vi "Begin.vi"(8 "error in":errorcluster) -> (0 "error out":errorcluster)   [LabVIEW 2016]
doc: "Called before other user functions, this VI is expected to open initial I/O refnums, load in file data, and do all program initialization. Notice that the <B>error out</B> terminal is simply used for data flow. Wiring it to other structures or subVIs ensures that this VI runs first."
uses:
  <vilib>/Rock Robotics/WPI/SafetyOutput/WPI_SafetyOutputConfigMenu.ctl
  <vilib>/Rock Robotics/WPI/DriverStation/WPI_DriverStationRobotMode2.ctl
  <vilib>/Rock Robotics/WPI/Joystick/WPI_JoystickDeviceEnum.ctl
  <vilib>/Rock Robotics/SystemInterfaces/AI/FPGA_AIChannel.ctl
  <vilib>/Rock Robotics/SystemInterfaces/DIO/FPGA_DIOChannel.ctl
  <vilib>/Rock Robotics/SystemInterfaces/i2clib/i2c_bus.ctl
  <vilib>/Rock Robotics/SystemInterfaces/DIO/FPGA_DIOPWMChannel.ctl
  <vilib>/Rock Robotics/SystemInterfaces/DIO/FPGA_DIORelayChannel.ctl
  <vilib>/Rock Robotics/WPI/Relay/WPI_RelayDirection.ctl
  <vilib>/Rock Robotics/WPI/Solenoid/WPI_SolenoidChannel.ctl
  Libraries/TalonSRX/TalonSRX/WPI_CANTalonSRX_APIControlMode.ctl
  Libraries/TalonSRX/TalonSRX/WPI_CANTalonSRX_APIFeedbackSelect.ctl
  Robot Global Data.vi
  <vilib>/Rock Robotics/Network Tables/NT Write String Array.vi
  <vilib>/Rock Robotics/WPI/MotorControl/WPI_MotorControlOpen SPARK.vi
  <vilib>/Rock Robotics/WPI/Solenoid/WPI_SolenoidOpenDouble.vi
  <vilib>/Rock Robotics/WPI/RobotDrive/WPI_RobotDriveOpen2MotorWithExistingMotors.vi
  Libraries/navX Library v2/navX Library v2.lvlib
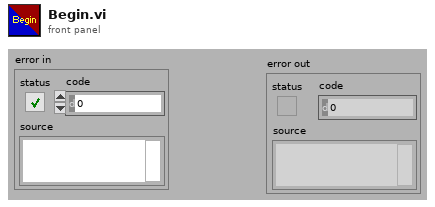
[diagram p1: front panel]
types:
  T1 = typedef "WPI_SolenoidChannel.ctl" = enum8{"Solenoid 0", "Solenoid 1", "Solenoid 2", "Solenoid 3", "Solenoid 4", "Solenoid 5", "Solenoid 6", "Solenoid 7", "Invalid"}
  T2 = typedef "WPI_CANTalonSRX_APIFeedbackSelect.ctl" = enum16{"Digital Quadrature Encoder", "Analog Potentiometer", "Analog Encoder", "Count on Quad-A (Rising-Edge)", "Count on Quad-A (Falling-Edge)", "CTR Magnetic Enc (Absolute)", "CTR Magnetic Enc (Relative)", "Pulse Width"}
  T3 = typedef "WPI_CANTalonSRX_APIControlMode.ctl" = enum8{"Percent VBus", "Speed", "Position", "Slave", "Unchanged / Invalid", "Voltage Compensation", "Current", "Motion Profile", "Motion Magic"}
  T4 = typedef "WPI_RelayDirection.ctl" = enum16{"Both directions", "Forward only", "Reverse only"}
  T5 = typedef "FPGA_DIORelayChannel.ctl" = enum8{"Relay 0", "Relay 1", "Relay 2", "Relay 3", "Invalid"}
  T6 = typedef "FPGA_DIOPWMChannel.ctl" = enum8{"PWM 0", "PWM 1", "PWM 2", "PWM 3", "PWM 4", "PWM 5", "PWM 6", "PWM 7", "PWM 8", "PWM 9", "PWM MXP 0", "PWM MXP 1", "PWM MXP 2", "PWM MXP 3", "PWM MXP 4", "PWM MXP 5", "PWM MXP 6", "PWM MXP 7", "PWM MXP 8", "PWM MXP 9", "Invalid"}
  T7 = typedef "FPGA_AIChannel.ctl" = enum8{"AI 0", "AI 1", "AI 2", "AI 3", "AI MXP 0", "AI MXP 1", "AI MXP 2", "AI MXP 3", "Invalid"}
  T8 = typedef "FPGA_DIOChannel.ctl" = enum8{"DIO 0", "DIO 1", "DIO 2", "DIO 3", "DIO 4", "DIO 5", "DIO 6", "DIO 7", "DIO 8", "DIO 9", "DIO MXP 0", "DIO MXP 1", "DIO MXP 2", "DIO MXP 3", "DIO MXP 4", "DIO MXP 5", "DIO MXP 6", "DIO MXP 7", "DIO MXP 8", "DIO MXP 9", "DIO MXP 10", "DIO MXP 11", "DIO MXP 12", "DIO MXP 13", "DIO MXP 14", "DIO MXP 15", "SPI Port CS1", "SPI Port CS2", "SPI Port CS3", "SPI Port MISO", "SPI Port MOSI", "Invalid"}
  T9 = typedef "WPI_JoystickDeviceEnum.ctl" = enum16{"USB 0", "USB 1", "USB 2", "USB 3", "USB 4", "USB 5"}
  T10 = typedef "i2c_bus.ctl" = enum16{"I2C On-Board", "I2C MXP", "Invalid"}
  T11 = typedef "WPI_DriverStationRobotMode2.ctl" = enum16{"Autonomous Disabled", "Autonomous Enabled", "Teleop Disabled", "Teleop Enabled", "Disconnected", "Finish", "Test Disabled", "Test Enabled", "Emergency Stopped"}
  T12 = typedef "WPI_SafetyOutputConfigMenu.ctl" = enum16{"Enable", "Disable"}
  T13 = typedef "WPI_MotorControlDeviceRef.ctl" = cluster{"DeviceStatus":errorcluster, "Type":T14, "PWM":cluster{"PWM Channel":T6, "DeadBand":T15}, "CAN":cluster{"Device Number":u8, "SetOutput VI Ref":variant, "GetOutput VI Ref":variant, "Enable VI Ref":variant, "Disable VI Ref":variant, "Data":variant}, "Invert":bool}
  T14 = typedef "WPI_MotorControlType.ctl" = enum16{"PWM", "CAN"}
  T15 = typedef "WPI_PWMDeadband.ctl" = cluster{"Name":string, "maxPositivePwm":i32, "minPositivePwm":i32, "centerPwm":i32, "maxNegativePwm":i32, "minNegativePwm":i32, "angularRange":u16}
  T16 = typedef "WPI_AnalogChannelDevRef.ctl" = cluster{"DevStatus":errorcluster, "Analog Channel":T7}
  T17 = typedef "WPI_DigitalInputDevRef.ctl" = cluster{"DevStatus":errorcluster, "DIO Channel":T8}
  T18 = typedef "WPI_JoystickDevRef.ctl" = cluster{"Device":T9}
  T19 = typedef "navX Library v2.lvlib/Z900_navX_DeviceTypeDef.ctl" = cluster{"Interface":cluster{"Protocol":T20, "Update Rate (4Hz-100Hz)":u8, "navX Open TypeDef":variant}, "Notify Packet":refnum<notifier>, "Loop VI Refnum":refnum<vi>, "Ready to Close Occurrence Refnum":refnum<k4>}
  T20 = typedef "navX Library v2.lvlib/Z900_navX_ProtocolTypeDef.ctl" = enum16{"SERIAL", "I2C", "SPI"}
  T21 = typedef "WPI_SolenoidDevRef.ctl" = cluster{"DevStatus":errorcluster, "Pneumatics Control Module":u8, "Forward Solenoid Channel":T1, "Reverse Solenoid Channel":T1}
  T22 = typedef "WPI_RelayDevRef.ctl" = cluster{"DevStatus":errorcluster, "Relay Channel":T5, "Relay Direction":T4}
  T23 = typedef "WPI_RobotDriveDevRef.ctl" = cluster{"DevStatus":errorcluster, "Motors[]":T13[], "Square Inputs":bool, "Max Output":dbl}
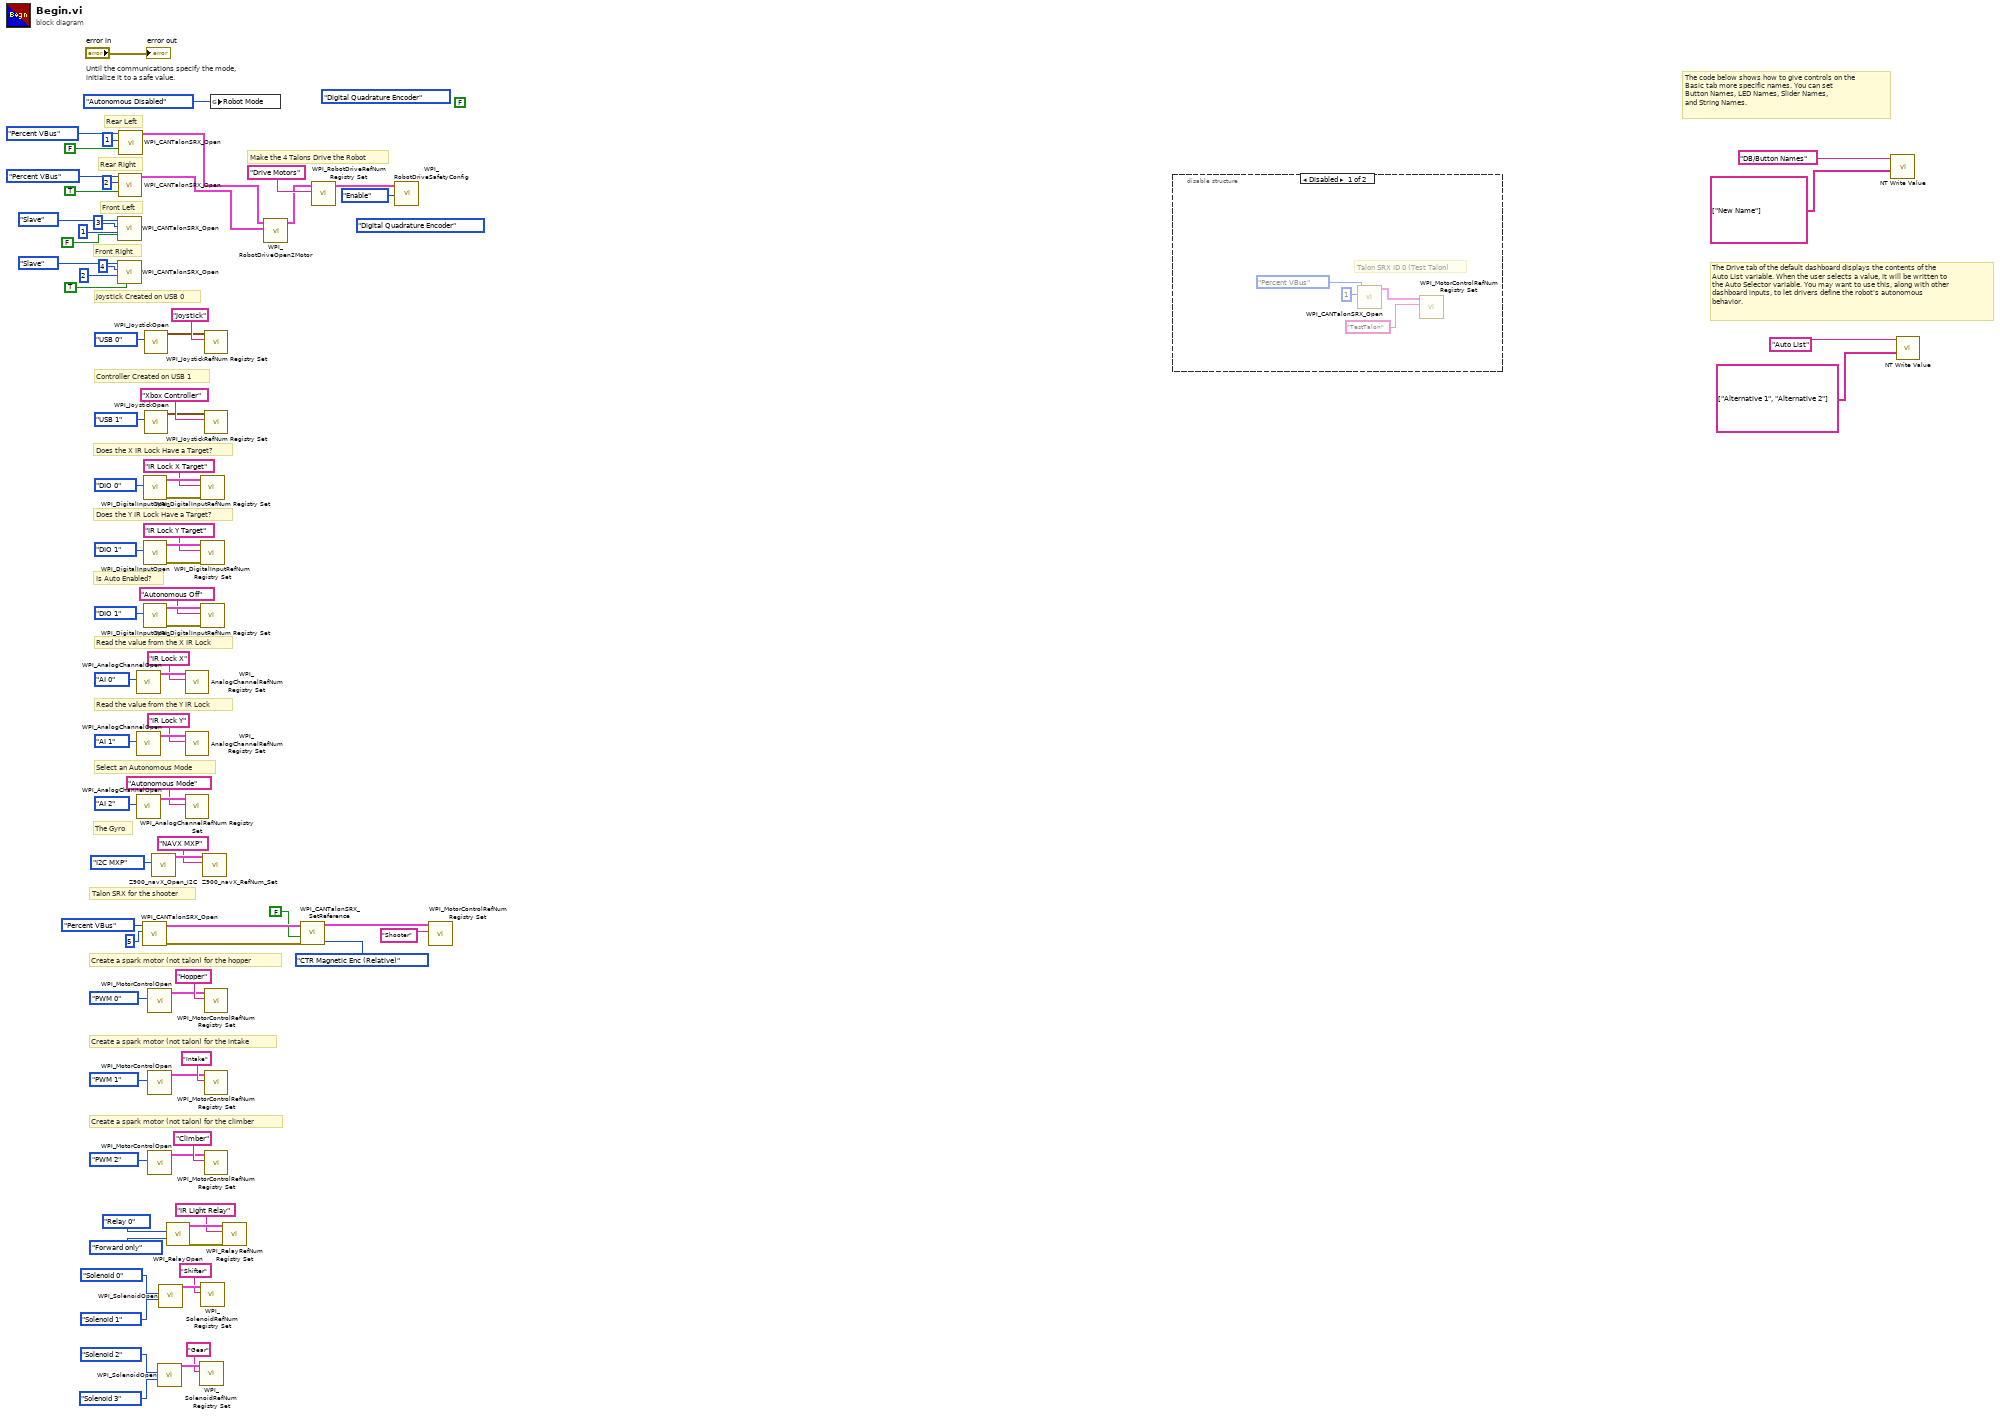
[diagram p0: block diagram]
diagram:
  (unwired) WPI_CANTalonSRX_APIFeedbackSelect."Digital Quadrature Encoder" ("Feedback Reference")
  (unwired) FALSE ("Reverse Feedback Sensor")
  (unwired) WPI_CANTalonSRX_APIFeedbackSelect."Digital Quadrature Encoder" ("Feedback Reference")
  # "Create a spark motor (not talon) for the climber"
  # "Create a spark motor (not talon) for the intake"
  # "Create a spark motor (not talon) for the hopper"
  # "Talon SRX for the shooter"
  # "The Gyro"
  # "Select an Autonomous Mode"
  # "Is Auto Enabled?"
  # "Read the value from the Y IR Lock"
  # "Read the value from the X IR Lock"
  # "Does the Y IR Lock Have a Target?"
  # "Does the X IR Lock Have a Target?"
  # "Make the 4 Talons Drive the Robot"
  # "Front Right"
  # "Front Left"
  # "Rear Right"
  # "Rear Left"
  # "Controller Created on USB 1"
  # "Joystick Created on USB 0"
  # "The Drive tab of the default dashboard displays the contents of the\nAuto List variable. When the user selects a value, it will be written to\nthe Auto Selector variable. You may want to use this, along with other\ndashboard inputs, to let drivers define the robot's autonomous\nbehavior."
  # "The code below shows how to give controls on the\nBasic tab more specific names. You can set\nButton Names, LED Names, Slider Names,\nand String Names."
  # "Until the communications specify the mode,\ninitialize it to a safe value."
  n1 = call "WPI_CANTalonSRX_Open.vi"("Invert"=FALSE, "Master Device Number"=u8 1, "Device Number"=u8 3, "Control Mode"=WPI_CANTalonSRX_APIControlMode."Slave") -> ()  [unwired: 6 in, 2 out]
  n2 = call "WPI_CANTalonSRX_Open.vi"("Invert"=TRUE, "Master Device Number"=u8 2, "Device Number"=u8 4, "Control Mode"=WPI_CANTalonSRX_APIControlMode."Slave") -> ()  [unwired: 6 in, 2 out]
  n3 = call "WPI_CANTalonSRX_Open.vi"("Invert"=TRUE, "Device Number"=u8 2, "Control Mode"=WPI_CANTalonSRX_APIControlMode."Percent VBus") -> ("CAN Talon SRX Ref"=w6:T13)  [unwired: 7 in, 1 out]
  n4 = call "WPI_CANTalonSRX_Open.vi"("Invert"=FALSE, "Device Number"=u8 1, "Control Mode"=WPI_CANTalonSRX_APIControlMode."Percent VBus") -> ("CAN Talon SRX Ref"=w7:T13)  [unwired: 7 in, 1 out]
  n5 = call <vilib>:"WPI_AnalogChannelOpen.vi"("Analog Channel"=FPGA_AIChannel."AI 0") -> ("AIDeviceRef"=w74:T16)  [unwired: 9 in, 1 out]
  n6 = call <vilib>:"WPI_AnalogChannelOpen.vi"("Analog Channel"=FPGA_AIChannel."AI 1") -> ("AIDeviceRef"=w53:T16)  [unwired: 9 in, 1 out]
  n7 = call <vilib>:"WPI_AnalogChannelOpen.vi"("Analog Channel"=FPGA_AIChannel."AI 2") -> ("AIDeviceRef"=w46:T16)  [unwired: 9 in, 1 out]
  n8 = call "WPI_CANTalonSRX_Open.vi"("Device Number"=u8 5, "Control Mode"=WPI_CANTalonSRX_APIControlMode."Percent VBus") -> ("error out"=w8:errorcluster, "CAN Talon SRX Ref"=w12:T13)  [unwired: 8 in]
  n9 = call <vilib>:"WPI_DigitalInputOpen.vi"("DIO Channel"=FPGA_DIOChannel."DIO 0") -> ("error out"=w71:errorcluster, "DigitalInputDevRef"=w70:T17)  [unwired: 9 in]
  n10 = call <vilib>:"WPI_DigitalInputOpen.vi"("DIO Channel"=FPGA_DIOChannel."DIO 1") -> ("error out"=w57:errorcluster, "DigitalInputDevRef"=w56:T17)  [unwired: 9 in]
  n11 = call <vilib>:"WPI_DigitalInputOpen.vi"("DIO Channel"=FPGA_DIOChannel."DIO 1") -> ("error out"=w50:errorcluster, "DigitalInputDevRef"=w49:T17)  [unwired: 9 in]
  n12 = call <vilib>:"WPI_JoystickOpen.vi"("JoystickDevice"=WPI_JoystickDeviceEnum."USB 0") -> ("JoystickDevRef"=w81:T18)  [unwired: 10 in]
  n13 = call <vilib>:"WPI_JoystickOpen.vi"("JoystickDevice"=WPI_JoystickDeviceEnum."USB 1") -> ("JoystickDevRef"=w63:T18)  [unwired: 10 in]
  n14 = call-poly <vilib>:"WPI_MotorControlOpen.vi"("PWM Channel"=FPGA_DIOPWMChannel."PWM 0") -> ("MotorControlDeviceRef"=w39:T13)  [unwired: 9 in, 1 out]
  n15 = call-poly <vilib>:"WPI_MotorControlOpen.vi"("PWM Channel"=FPGA_DIOPWMChannel."PWM 1") -> ("MotorControlDeviceRef"=w36:T13)  [unwired: 9 in, 1 out]
  n16 = call-poly <vilib>:"WPI_MotorControlOpen.vi"("PWM Channel"=FPGA_DIOPWMChannel."PWM 2") -> ("MotorControlDeviceRef"=w33:T13)  [unwired: 9 in, 1 out]
  n17 = call "Z900_navX_Open_I2C.vi"("I2C Bus"=i2c_bus."I2C MXP") -> ("navX Device"=w67:T19)  [unwired: 9 in, 1 out]
  n18 = call-poly <vilib>:"WPI_SolenoidOpen.vi"("Reverse Solenoid Channel"=WPI_SolenoidChannel."Solenoid 3", "Forward Solenoid Channel"=WPI_SolenoidChannel."Solenoid 2" ("Solenoid Channel")) -> ("SolenoidDevRef"=w4:T21)  [unwired: 8 in, 1 out]
  n19 = call-poly <vilib>:"WPI_SolenoidOpen.vi"("Reverse Solenoid Channel"=WPI_SolenoidChannel."Solenoid 1", "Forward Solenoid Channel"=WPI_SolenoidChannel."Solenoid 0" ("Solenoid Channel")) -> ("SolenoidDevRef"=w26:T21)  [unwired: 8 in, 1 out]
  n20 = call <vilib>:"WPI_RelayOpen.vi"("Relay Direction"=WPI_RelayDirection."Forward only", "Relay Channel"=FPGA_DIORelayChannel."Relay 0") -> ("error out"=w30:errorcluster, "RelayDevRef"=w31:T22)  [unwired: 8 in]
  n21 = call <vilib>:"WPI_AnalogChannelRefNum Registry Set.vi"("refnum name"="IR Lock X", "AIDeviceRef"=w74) -> ()  [unwired: 8 in, 2 out]
  n22 = call <vilib>:"WPI_AnalogChannelRefNum Registry Set.vi"("refnum name"="IR Lock Y", "AIDeviceRef"=w53) -> ()  [unwired: 8 in, 2 out]
  n23 = call <vilib>:"WPI_AnalogChannelRefNum Registry Set.vi"("refnum name"="Autonomous Mode", "AIDeviceRef"=w46) -> ()  [unwired: 8 in, 2 out]
  n24 = call <vilib>:"WPI_SolenoidRefNum Registry Set.vi"("refnum name"="Gear", "SolenoidDevRef"=w4) -> ()  [unwired: 8 in, 2 out]
  n25 = call <vilib>:"WPI_DigitalInputRefNum Registry Set.vi"("error in (no error)"=w71, "refnum name"="IR Lock X Target", "DigitalInputDevRef"=w70) -> ()  [unwired: 7 in, 2 out]
  n26 = call <vilib>:"WPI_DigitalInputRefNum Registry Set.vi"("error in (no error)"=w57, "refnum name"="IR Lock Y Target", "DigitalInputDevRef"=w56) -> ()  [unwired: 7 in, 2 out]
  n27 = call <vilib>:"WPI_DigitalInputRefNum Registry Set.vi"("error in (no error)"=w50, "refnum name"="Autonomous Off", "DigitalInputDevRef"=w49) -> ()  [unwired: 7 in, 2 out]
  n28 = call <vilib>:"WPI_SolenoidRefNum Registry Set.vi"("refnum name"="Shifter", "SolenoidDevRef"=w26) -> ()  [unwired: 8 in, 2 out]
  n29 = call "Z900_navX_RefNum_Set.vi"("refnum name"="NAVX MXP", "navX Device"=w67) -> ()  [unwired: 8 in, 2 out]
  n30 = call <vilib>:"WPI_JoystickRefNum Registry Set.vi"("refnum name"="Joystick", "JoystickDevRef"=w81) -> ()  [unwired: 8 in, 2 out]
  n31 = call <vilib>:"WPI_JoystickRefNum Registry Set.vi"("refnum name"="Xbox Controller", "JoystickDevRef"=w63) -> ()  [unwired: 8 in, 2 out]
  n32 = call <vilib>:"WPI_MotorControlRefNum Registry Set.vi"("refnum name"="Hopper", "MotorControlDevRef"=w39) -> ()  [unwired: 8 in, 2 out]
  n33 = call <vilib>:"WPI_MotorControlRefNum Registry Set.vi"("refnum name"="Intake", "MotorControlDevRef"=w36) -> ()  [unwired: 8 in, 2 out]
  n34 = call <vilib>:"WPI_MotorControlRefNum Registry Set.vi"("refnum name"="Climber", "MotorControlDevRef"=w33) -> ()  [unwired: 8 in, 2 out]
  n35 = global write "Robot Global Data.vi" "Robot Mode"(WPI_DriverStationRobotMode2."Autonomous Disabled" ("Robot Mode")) -> ()
  n36 = call <vilib>:"WPI_RelayRefNum Registry Set.vi"("error in (no error)"=w30, "refnum name"="IR Light Relay", "RelayDevRef"=w31) -> ()  [unwired: 7 in, 2 out]
  n37 = call-poly <vilib>:"WPI_RobotDriveOpen2Motor.vi"("Right Motor Dev Ref"=w6, "Left Motor Dev Ref"=w7) -> ("RobotDriveDevRef"=w5:T23)  [unwired: 8 in, 1 out]
  n38 = call "WPI_CANTalonSRX_SetReference.vi"("error in (no error)"=w8, "Reverse Feedback Sensor"=FALSE, "Feedback Reference"=WPI_CANTalonSRX_APIFeedbackSelect."CTR Magnetic Enc (Relative)", "CAN Talon SRX Ref"=w12) -> ("CAN Talon SRX Ref"=w11:T13)  [unwired: 6 in, 1 out]
  n39 = call <vilib>:"WPI_RobotDriveRefNum Registry Set.vi"("refnum name"="Drive Motors", "RobotDriveDevRef"=w5) -> ("RobotDriveDevRef"=w85:T23)  [unwired: 2 in, 7 out]
  n40 = call <vilib>:"WPI_RobotDriveSafetyConfig.vi"("mode"=WPI_SafetyOutputConfigMenu."Enable", "RobotDriveDevRef"=w85) -> ()  [unwired: 8 in, 2 out]
  n41 = call <vilib>:"WPI_MotorControlRefNum Registry Set.vi"("refnum name"="Shooter", "MotorControlDevRef"=w11) -> ()  [unwired: 8 in, 2 out]
  n42 = disable-structure shown="Disabled" {
    frame Disabled {
      # "Talon SRX ID 0 (Test Talon)"
      n43 = call "WPI_CANTalonSRX_Open.vi"("Device Number"=u8 1, "Control Mode"=WPI_CANTalonSRX_APIControlMode."Percent VBus") -> ("CAN Talon SRX Ref"=w88:T13)  [unwired: 8 in, 1 out]
      n44 = call <vilib>:"WPI_MotorControlRefNum Registry Set.vi"("refnum name"="TestTalon", "MotorControlDevRef"=w88) -> ()  [unwired: 8 in, 2 out]
    }
    frame Enabled {
    }
  }
  n45 = call-poly <vilib>:"NT Write Value.vi"("String Array"=string[] ["New Name"], "Name"="DB/Button Names") -> ()  [unwired: 9 in, 1 out]
  n46 = call-poly <vilib>:"NT Write Value.vi"("String Array"=string[] ["Alternative 1", "Alternative 2"], "Name"="Auto List") -> ()  [unwired: 9 in, 1 out]
  "error out" <- "error in"
